vi "ModelParameterValueUpdateFromFile.vi"(9 "Target":string, 10 "parameter_files":string[](array[string]), 11 "ModelManager in":T1) -> (0 "error out":errorcluster, 1 "Target out":string, 2 "parameter_files out":string[](array[string]))   [LabVIEW 2015, in "MiscHelperVIs.lvlib"]
uses:
  MiscHelperVIs.lvlib
  <vilib>/NI Veristand/Execution/ModelManager/ModelManagerAPI.ctl
  NationalInstruments.VeriStand.ClientAPI
  NationalInstruments.VeriStand
  <vilib>/NI Veristand/Execution/ModelManager/NI_VS ModelManager ExecutionAPI.lvlib
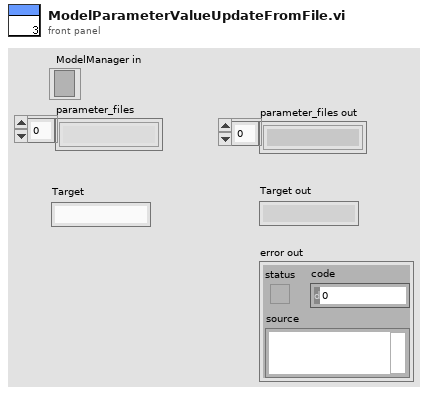
[diagram p1: front panel]
types:
  T1 = typedef "NI_VS ModelManager ExecutionAPI.lvlib/ModelManagerAPI.ctl" = refnum<k24>
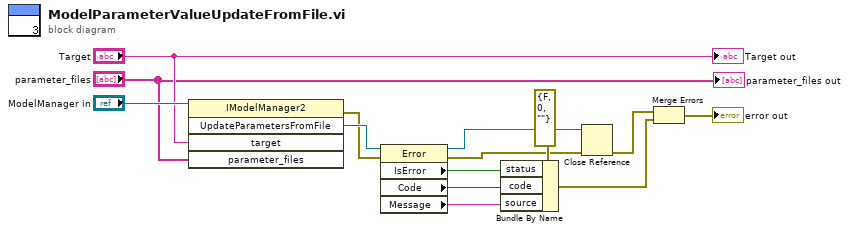
[diagram p0: block diagram]
diagram:
  n1 = invoke class="IModelManager2" method="UpdateParametersFromFile"(reference="ModelManager in", "target"="Target", "parameter_files"="parameter_files") -> (error out=w6:errorcluster, "UpdateParametersFromFile"=w12:refnum<k24>)  [unwired: 2 in, 3 out]
  n2 = property class="Error"(reference=w12, error in=w6) -> (reference out=w4:refnum<k24>, error out=w5:errorcluster, "IsError"=w8:bool, "Code"=w9:u32, "Message"=w10:string)
  n3 = Bundle By Name(cluster=errorcluster {"status"=FALSE, "code"=0, "source"=""} ("error in (no error)"), "status"=w8, "code"=w9, "source"=w10) -> (w2:errorcluster)
  n4 = Close Reference(reference=w4, error in (no error)=w5) -> (error out=w3:errorcluster)
  n5 = Merge Errors(w3, w2) -> (→"error out":errorcluster)
  "Target out" <- "Target"
  "parameter_files out" <- "parameter_files"
